vi "Set_RegData_Value.vi"(8 "error in (no error)":errorcluster, 10 "New Val":string, 11 "RegData_String in":refnum<class "IB_RegData_String.lvclass">) -> (0 "error out":errorcluster, 2 "Val":string, 3 "RegData_String out":refnum<class "IB_RegData_String.lvclass">)   [LabVIEW 2020, in "IB_RegData_String.lvclass"]
uses:
  <vilib>/AppBuilder/IB_Classes/RegData/RegData_String/IB_RegData_String.lvclass
  <vilib>/AppBuilder/IB_Classes/RegData/RegData_String/IB_RegData_String.lvclass/IB_RegData_String.ctl
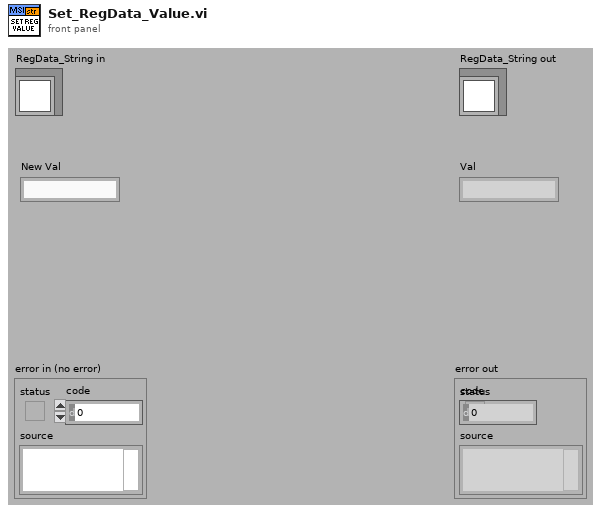
[diagram p1: front panel]
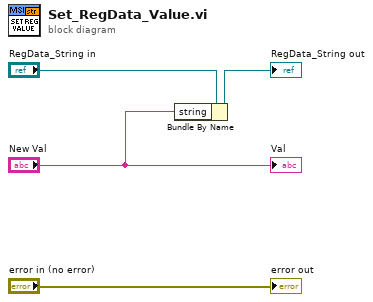
[diagram p0: block diagram]
diagram:
  n1 = Bundle By Name(cluster="RegData_String in", "string"="New Val") -> (→"RegData_String out":refnum<class "IB_RegData_String.lvclass">)
  "error out" <- "error in (no error)"
  "Val" <- "New Val"
